vi "VarToData - Live.vi"(11 "data":variant) -> (1 "param":u32, 2 "Command":string, 3 "cam0 Session":T1)   [LabVIEW 2020]
uses:
  <vilib>/userDefined/High Color/IMAQdx.ctl
  _controls/xiCam.ctl
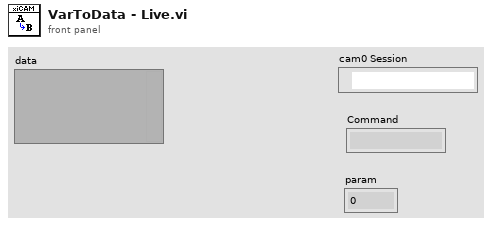
[diagram p1: front panel]
types:
  T1 = typedef "IMAQdx.ctl" = refnum<k21>
  T2 = typedef "xiCam.ctl" = cluster{"Exposure Time (ms)":u32, "cam0 Session":T1, "Camera ROI":cluster{"Width":u32, "Height":u32, "Offset X":u32, "Offset Y":u32}, "Command":string}
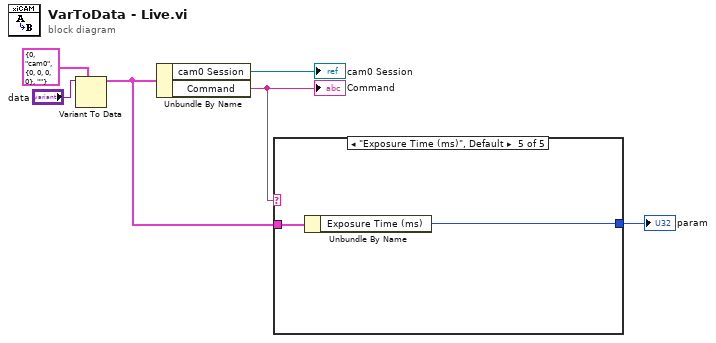
[diagram p0: block diagram]
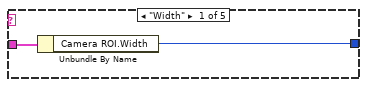
[diagram p2: hidden frame]
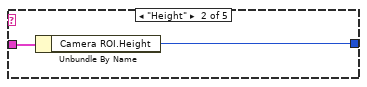
[diagram p3: hidden frame]
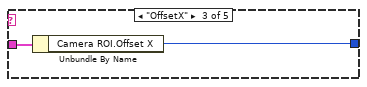
[diagram p4: hidden frame]
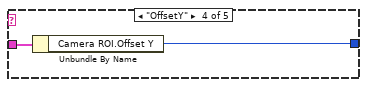
[diagram p5: hidden frame]
diagram:
  n1 = Variant To Data(type=T2 {"Exposure Time (ms)"=0, "cam0 Session"="cam0", "Camera ROI"={"Width"=0, "Height"=0, "Offset X"=0, "Offset Y"=0}, "Command"=""} ("Camera Controls"), Variant="data") -> (data=w2:T2)  [unwired: 1 in, 1 out]
  n2 = Unbundle By Name(w2) -> ("cam0 Session"=→"cam0 Session":T1, "Command"=w3:string)
  "Command" <- w3
  n3 = case shown="\"Exposure Time (ms)\", Default" w3 {
    tunnel: w2 -> [w8 w10 w12 w14 w15]
    tunnel: [w7 w9 w11 w13 w16] -> w1
    frame "Width" {
      n4 = Unbundle By Name(w8) -> ("Camera ROI.Width"=w7:u32)
    }
    frame "Height" {
      n5 = Unbundle By Name(w10) -> ("Camera ROI.Height"=w9:u32)
    }
    frame "OffsetX" {
      n6 = Unbundle By Name(w12) -> ("Camera ROI.Offset X"=w11:u32)
    }
    frame "OffsetY" {
      n7 = Unbundle By Name(w14) -> ("Camera ROI.Offset Y"=w13:u32)
    }
    frame "Exposure Time (ms)", Default {
      n8 = Unbundle By Name(w15) -> ("Exposure Time (ms)"=w16:u32)
    }
  }
  "param" <- w1
